vi "FRIC_navX_Internal_I2C_ProcessingLoop.vi"(7 "Device Number":T2, 10 "I2C Bus":T1=enum."I2C MXP", 11 "Rate (4Hz-200Hz)":u8=50 min=4 max=200) -> ()   [LabVIEW 2016]
doc: "This navX VI handles the reading/writing for the navX. All of the good stuff is in here.\nTHIS VI SHOULD NOT BE CALLED BY THE USER!"
uses:
  <vilib>/Rock Robotics/SystemInterfaces/i2clib/i2c_bus.ctl
  TypeDefs/Z900_navX_ProtocolTypeDef.ctl
  navX Library v2.lvlib
  TypeDefs/FRIC_navX_ProcessingLoopStatesTypeDef_I2C.ctl
  TypeDefs/Z900_navX_IntegrationControlRegisters.ctl
  TypeDefs/Z900_navX_ActionTypeDef.ctl
  TypeDefs/Z900_navX_NotifyPacketTypeDef.ctl
  TypeDefs/FRIC_navX_I2C Process Loop TypeDef.ctl
  TypeDefs/Flags/Z900_navX_Flags_CapabilityTypeDef.ctl
  TypeDefs/Z900_navX_DeviceRegisters.ctl
  <vilib>/Rock Robotics/SystemInterfaces/spilib/spi_bus.ctl
  <vilib>/Rock Robotics/WPI/SPI/WPI_SPIDevRef.ctl
  <vilib>/Rock Robotics/WPI/SerialPort/WPI_SerialPortRef.ctl
  TypeDefs/Z900_navX_SerialStreamTypeDef.ctl
  TypeDefs/FRIC_navX_DeviceNumbersTypeDef.ctl
  <vilib>/Rock Robotics/WPI/SerialPort/WPI_SerialPort.ctl
  <vilib>/Platform/TimedLoop/XDataNode/wakeup.ctl
  <vilib>/Platform/TimedLoop/XDataNode/XDNodeRunTimeDep.lvlib
  <vilib>/Platform/TimedLoop/XDataNode/nitl_modes.ctl
  <vilib>/Platform/TimedLoop/XDataNode/timing_clust.ctl
  <vilib>/Platform/TimedLoop/XDataNode/XDataNode.xnode
  <vilib>/ptbypt/NI_PtbyPt.lvlib
  TypeDefs/Z900_navX_DeviceTypeDef.ctl
panel:
  in  "Tab Control":enum32{"Page 1", "Page 2"}(tab)
  in  "Halt":bool
  out "Connected":bool
  out "error":errorcluster
  out "Loop Time":dbl
  out "Loop dt":i64
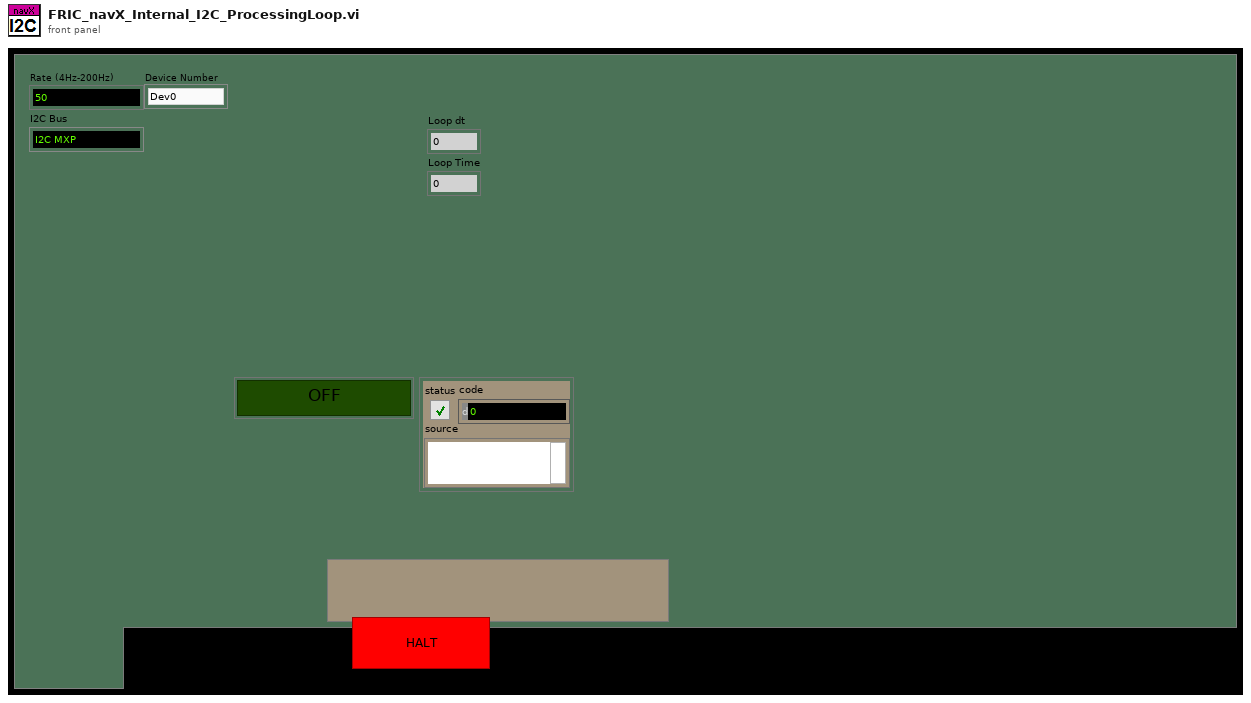
[diagram p1: front panel]
types:
  T1 = typedef "i2c_bus.ctl" = enum16{"I2C On-Board", "I2C MXP", "Invalid"}
  T2 = typedef "FRIC_navX_DeviceNumbersTypeDef.ctl" = enum16{"Dev0", "Dev1", "Dev2", "Dev3"}
  T3 = typedef "FRIC_navX_I2C Process Loop TypeDef.ctl" = cluster{"State Array":T4[], "error":errorcluster, "FPGA Cluster":cluster{"Last Valid FPGA Time":dbl, "Error Count":i32, "Initialized":bool}, "Device Info":T5, "I2CDevRef":cluster{"DevStatus":errorcluster, "Device Address":u8, "Handle":i32, "I2C Bus":T1}, "Registry":u8[], "Command Array":T7[], "Connected?":bool, "navX Device Memory Size":i32, "notification":T8, "Memory Size Set":bool, "SPIDevRef":T10, "navX Serial Open":cluster{"Stream Type":T12, "Serial Port":T13}, "SerialPortRef":T14, "Serial Read Buffer":string, "Serial Write Buffer":string[], "Device Number":T2, "navX SPI Open":cluster{"SPI Bus":T11, "Clock Rate (Hz)":dbl}, "Loop dt":i64, "current time":timestamp, "Loop Time":i64}
  T4 = typedef "FRIC_navX_ProcessingLoopStatesTypeDef_I2C.ctl" = enum16{"Process", "INI", "Check Packets Valid", "Close", "Flush Serial", "Generate Command", "Last Packet Valid", "Open", "Read", "Reset Serial", "Set Termination Char", "Update AE", "Wait", "Write", "Exit"}
  T5 = typedef "navX Library v2.lvlib/Z900_navX_DeviceTypeDef.ctl" = cluster{"Interface":cluster{"Protocol":T6, "Update Rate (4Hz-100Hz)":u8, "navX Open TypeDef":variant}, "Notify Packet":refnum<notifier>, "Loop VI Refnum":refnum<vi>, "Ready to Close Occurrence Refnum":refnum<k4>}
  T6 = typedef "navX Library v2.lvlib/Z900_navX_ProtocolTypeDef.ctl" = enum16{"SERIAL", "I2C", "SPI"}
  T7 = typedef "navX Library v2.lvlib/Z900_navX_IntegrationControlRegisters.ctl" = u8
  T8 = typedef "navX Library v2.lvlib/Z900_navX_NotifyPacketTypeDef.ctl" = cluster{"navX Action":T9, "Data":variant}
  T9 = typedef "navX Library v2.lvlib/Z900_navX_ActionTypeDef.ctl" = enum16{"None", "Halt", "Update Serial Protocol", "Zero-Yaw", "Zero-Displacement", "Zero-Velocity"}
  T10 = typedef "WPI_SPIDevRef.ctl" = cluster{"DevStatus":errorcluster, "Handle":i32, "SPI Bus":T11}
  T11 = typedef "spi_bus.ctl" = enum16{"SPI On-Board, CS0", "SPI On-Board, CS1", "SPI On-Board, CS2", "SPI On-Board, CS3", "SPI MXP", "Invalid"}
  T12 = typedef "navX Library v2.lvlib/Z900_navX_SerialStreamTypeDef.ctl" = enum16{"YRPH", "Quaterinons", "Gyro/Raw", "AHRS", "AHRSAndPositioning"}
  T13 = typedef "WPI_SerialPort.ctl" = enum16{"Onboard RS-232", "MXP TTL", "USB 1", "USB 2"}
  T14 = typedef "WPI_SerialPortRef.ctl" = cluster{"DevStatus":errorcluster, "Serial Port Name":refnum<visa-resource-name>}
  T15 = typedef "XDNodeRunTimeDep.lvlib/timing_clust.ctl" = cluster{"Expected End [f-1]":u64, "Actual End [f-1]":u64, "Finished Late? [f-1]":bool, "Expected End [i-1]":u64, "Actual End [i-1]":u64, "Finished Late? [i-1]":bool, "Expected Start [i]":u64, "Actual Start [i]":u64, "Expected Start [f]":u64, "Actual Start [f]":u64, "Source Name":string, "Structure Name":string, "Period":i64, "Deadline":i64, "Offset":i64, "Start":i64, "Priority":i32, "Timeout":i32, "Mode":T16, "Wakeup Reason":T17, "Error":errorcluster, "Source Type":string, "Secondary Source Type":string, "Global End Time":u64, "Global Start Time":u64, "Frame Duration":u64, "Iteration Duration":u64, "Assigned CPU":i32, "I/O Scan Engine Mode":u32}
  T16 = typedef "XDNodeRunTimeDep.lvlib/nitl_modes.ctl" = enum32{"No Change", "Process missed periods, maintain original phase", "Discard missed periods, maintain original phase", "Process missed periods, ignore original phase", "Discard missed periods, ignore original phase"}
  T17 = typedef "XDNodeRunTimeDep.lvlib/wakeup.ctl" = enum32{"Normal", "Aborted", "Asynchronous wakeup", "Timing source error", "Timed loop error", "Timeout"}
  T18 = typedef "Z900_navX_ActionTypeDef.ctl" = enum16{"None", "Halt", "Normal Read", "Update Serial Protocol", "Update Rate Htz", "Zero-Yaw", "Zero-Displacement", "Zero-Velocity"}
  T19 = typedef "navX Library v2.lvlib/Z900_navX_DeviceRegisters.ctl" = u8
  T20 = typedef "navX Library v2.lvlib/Z900_navX_Flags_CapabilityTypeDef.ctl" = u16
  T21 = cluster{"DevStatus":errorcluster, "Device Address":u8, "Handle":i32, "I2C Bus":T1}
  T22 = cluster{"Last Valid FPGA Time":dbl, "Error Count":i32, "Initialized":bool}
  T23 = typedef "WPI_I2CDevRef.ctl" = cluster{"DevStatus":errorcluster, "Device Address":u8, "Handle":i32, "I2C Bus":T1}
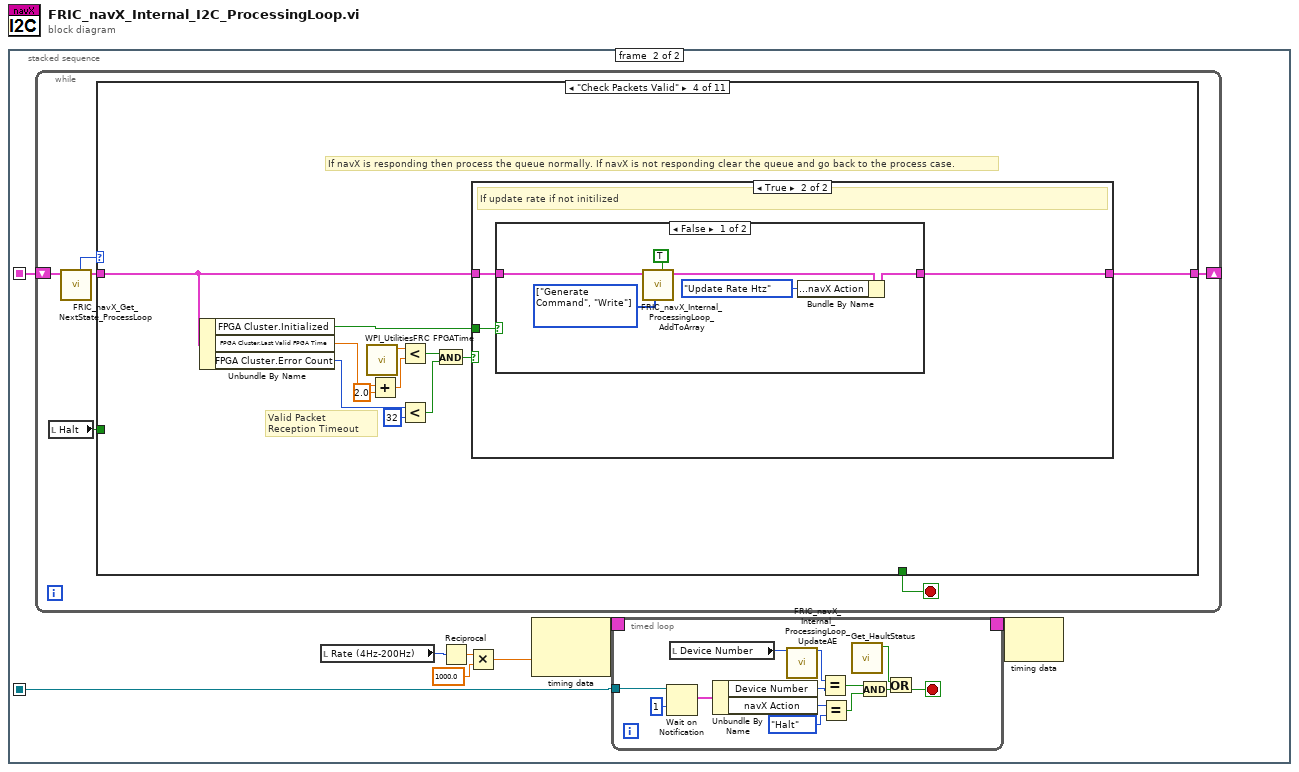
[diagram p0: block diagram]
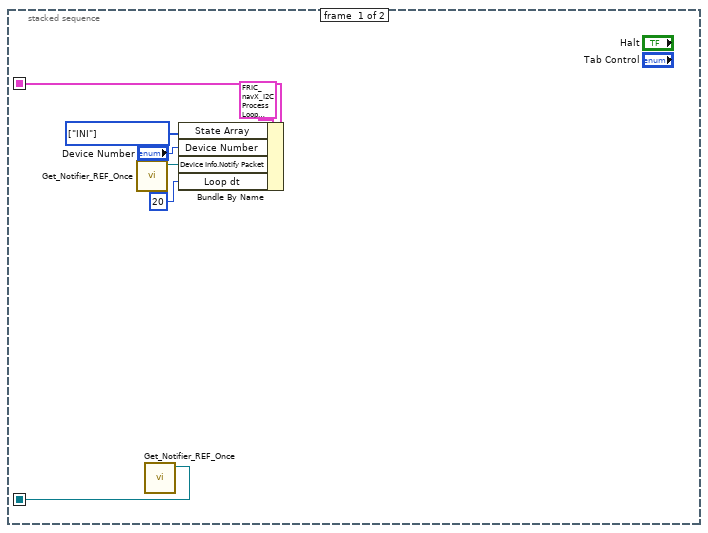
[diagram p2: hidden frame]
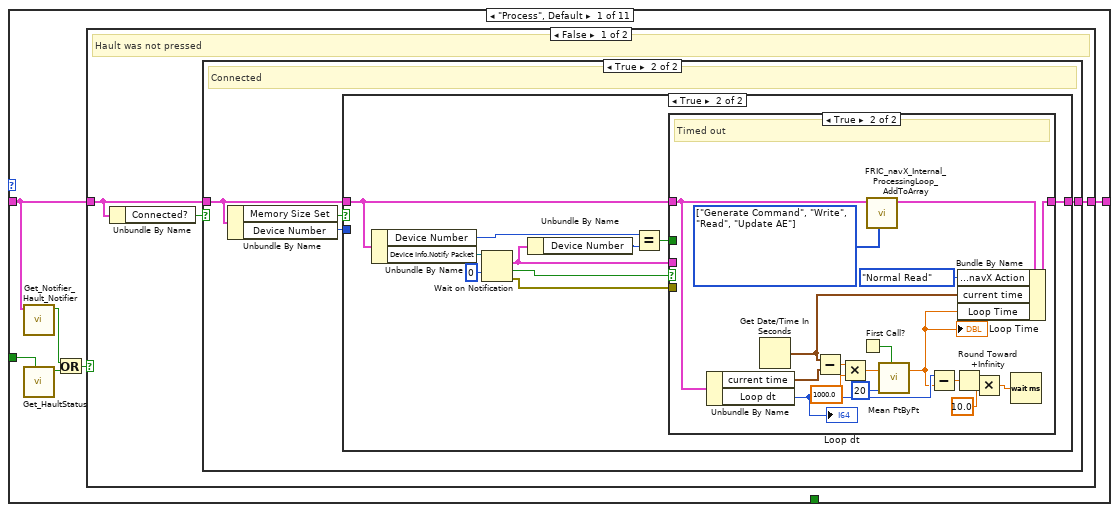
[diagram p3: hidden frame]
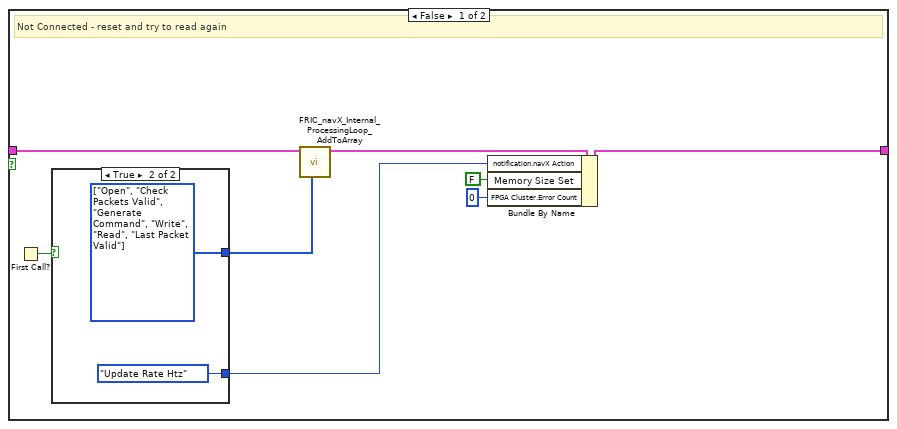
[diagram p4: hidden frame]
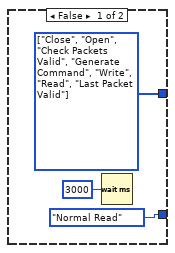
[diagram p5: hidden frame]
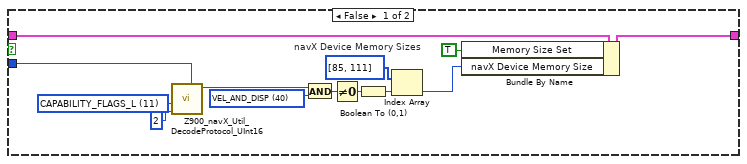
[diagram p6: hidden frame]
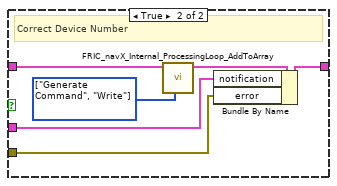
[diagram p8: hidden frame]
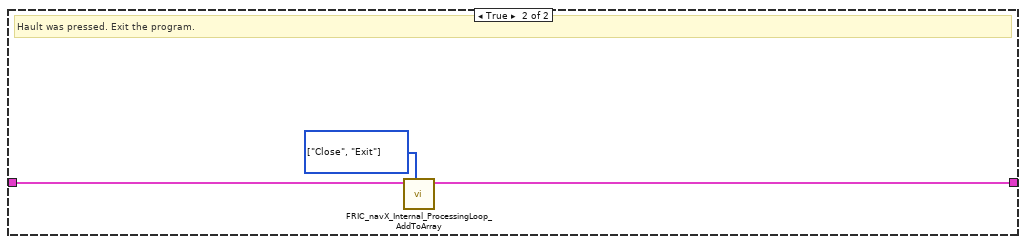
[diagram p9: hidden frame]
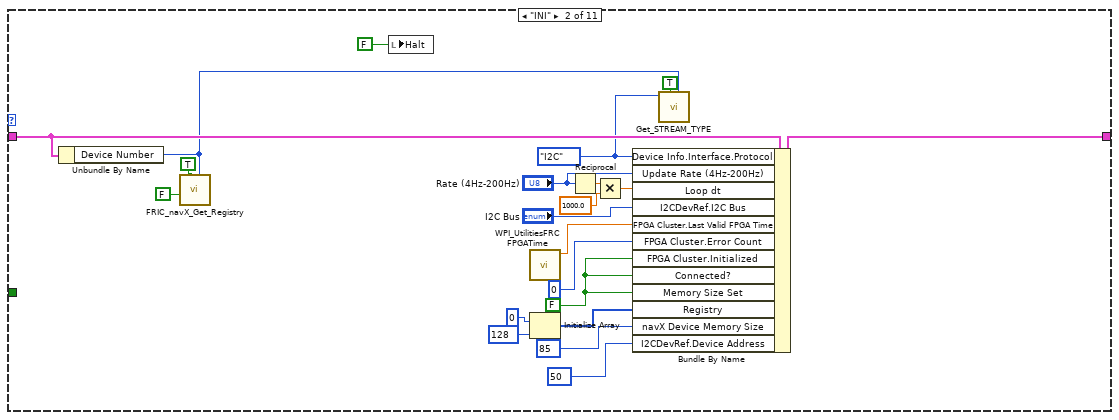
[diagram p10: hidden frame]
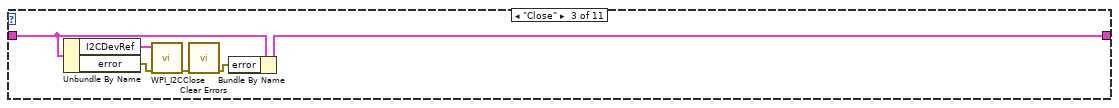
[diagram p11: hidden frame]
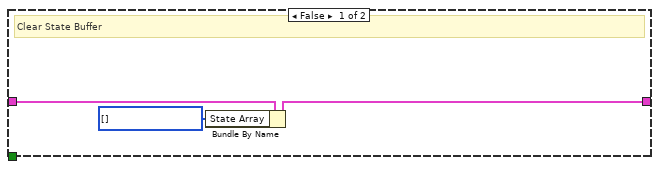
[diagram p12: hidden frame]
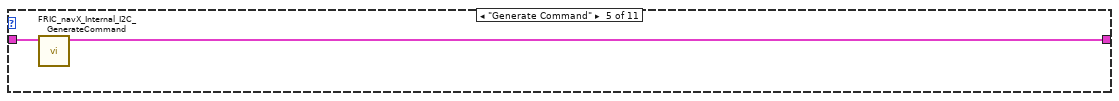
[diagram p14: hidden frame]
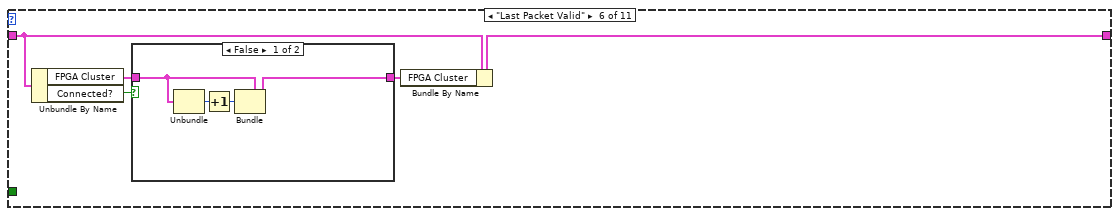
[diagram p15: hidden frame]
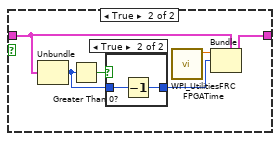
[diagram p16: hidden frame]
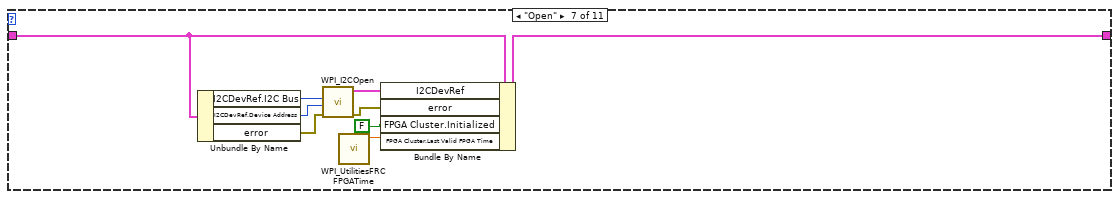
[diagram p18: hidden frame]
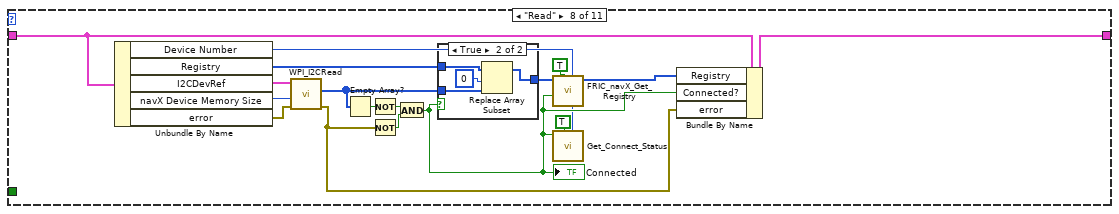
[diagram p19: hidden frame]
diagram:
  n1 = stacked-sequence {
    seq-local: [w7 _] -> [_ w15]
    seq-local: [w1 _] -> [_ w8]
    frame #0 {
      w5 = T4[] [enum."INI"] items=["Process", "INI", "Check Packets Valid", "Close", "Flush Serial", "Generate Command", "Last Packet Valid", "Open", "Read", "Reset Serial", "Set Termination Char", "Update AE", "Wait", "Write", "Exit"] ("State Array")
      n2 = call "Get_Notifier_REF_Once.vi"() -> ("notifier ref out"=w3:refnum<notifier>)  [unwired: 10 in, 1 out]
      n3 = call "Get_Notifier_REF_Once.vi"() -> ("notifier ref out"=w1:refnum<notifier>)  [unwired: 10 in, 1 out]
      n4 = Bundle By Name(cluster=T3 {"State Array"=[enum."INI", enum."Open"], "error"={"status"=FALSE, "code"=0, "source"=""}, "FPGA Cluster"={"Last Valid FPGA Time"=0.0, "Error Count"=0, "Initialized"=FALSE}, "Device Info"={"Interface"={"Protocol"=enum."SERIAL", "Update Rate (4Hz-100Hz)"=4, "navX Open TypeDef"=variant}, "Notify Packet"=refnum, "Loop VI Refnum"=refnum, "Ready to Close Occurrence Refnum"=refnum}, "I2CDevRef"={"DevStatus"={"status"=FALSE, "code"=0, "source"=""}, "Device Address"=0, "Handle"=0, "I2C Bus"=enum."Invalid"}, "Registry"=[], "Command Array"=[214, 32], "Connected?"=FALSE, "navX Device Memory Size"=85, "notification"={"navX Action"=enum."None", "Data"=variant}, "Memory Size Set"=FALSE, "SPIDevRef"={"DevStatus"={"status"=FALSE, "code"=0, "source"=""}, "Handle"=0, "SPI Bus"=enum."SPI On-Board, CS0"}, "navX Serial Open"={"Stream Type"=enum."YRPH", "Serial Port"=enum."Onboard RS-232"}, "SerialPortRef"={"DevStatus"={"status"=FALSE, "code"=0, "source"=""}, "Serial Port Name"=""}, "Serial Read Buffer"="", "Serial Write Buffer"=[], "Device Number"=enum."Dev0", "navX SPI Open"={"SPI Bus"=enum."SPI MXP", "Clock Rate (Hz)"=500000.0}, "Loop dt"=0, "current time"=timestamp(0 s since 1904-01-01), "Loop Time"=0} ("I2C Process Loop TypeDef"), "State Array"=w5, "Device Number"="Device Number", "Device Info.Notify Packet"=w3, "Loop dt"=i64 20) -> (w7:T3)
    }
    frame #1 {
      n5 = while {
        shift-right: [w35] -> _
        shift-left: w15 -> [w38]
        stop <- w39 stop-if-true
        n6 = local read "Halt"() -> (w34:bool)
        n7 = call "FRIC_navX_Get_NextState_ProcessLoop.vi"("I2C Process Loop TypeDef (in)"=w38) -> ("I2C Process Loop TypeDef (out)"=w37:T3, "Current State"=w36:T4)  [unwired: 9 in]
        n8 = case shown="\"Check Packets Valid\"" w36 {
          tunnel: [_ _ _ _ _ _ _ _ _ w233 _] -> w39
          tunnel: w37 -> [w44 w132 w146 w153 w175 w179 w201 w214 w231 w235 w243]
          tunnel: [w45 w138 w145 w154 w174 w178 w200 w213 w232 w235 w243] -> w35
          tunnel: w34 -> [w42 _ _ _ _ _ _ _ _ _ _]
          frame "Process", Default {
            n9 = call "Get_Notifier_Hault_Notifier.vi"("Process Loop TypeDef (in)"=w44) -> ("Hault Notifier"=w41:bool)  [unwired: 10 in]
            n10 = call "Get_HaultStatus.vi"("Update"=w42) -> ("Hault"=w40:bool)  [unwired: 10 in]
            n11 = Or(x=w41, y=w40) -> (x .or. y?=w43:bool)
            n12 = case shown="False" w43 {
              tunnel: [w48 w120] -> w45
              tunnel: w44 -> [w46 w121]
              frame False {
                # "Hault was not pressed"
                n13 = Unbundle By Name(w46) -> ("Connected?"=w47:bool)
                n14 = case shown="True" w47 {
                  tunnel: w46 -> [w56 w64]
                  tunnel: [w53 w65] -> w48
                  frame False {
                    # "Not Connected - reset and try to read again"
                    n15 = First Call?() -> (First Call?: T/F=w50:bool)
                    n16 = case shown="True" w50 {
                      tunnel: [w59 w61] -> w55
                      tunnel: [Z900_navX_ActionTypeDef."Normal Read" ("notification.navX Action") Z900_navX_ActionTypeDef."Update Rate Htz" ("notification.navX Action")] -> w49
                      frame False {
                        w59 = T4[] [enum."Close", enum."Open", enum."Check Packets Valid", enum."Generate Command", enum."Write", enum."Read", enum."Last Packet Valid"] items=["Process", "INI", "Check Packets Valid", "Close", "Flush Serial", "Generate Command", "Last Packet Valid", "Open", "Read", "Reset Serial", "Set Termination Char", "Update AE", "Wait", "Write", "Exit"]
                        n17 = Wait (ms)(milliseconds to wait=u32 3000) -> ()  [unwired: 1 out]
                      }
                      frame True {
                        w61 = T4[] [enum."Open", enum."Check Packets Valid", enum."Generate Command", enum."Write", enum."Read", enum."Last Packet Valid"] items=["Process", "INI", "Check Packets Valid", "Close", "Flush Serial", "Generate Command", "Last Packet Valid", "Open", "Read", "Reset Serial", "Set Termination Char", "Update AE", "Wait", "Write", "Exit"]
                      }
                    }
                    n18 = call "FRIC_navX_Internal_ProcessingLoop_AddToArray.vi"("States Array"=w55, "I2C Process Loop TypeDef (in)"=w56) -> ("I2C Process Loop TypeDef (out)"=w54:T3)  [unwired: 9 in]
                    n19 = Bundle By Name(cluster=w54, "notification.navX Action"=w49, "Memory Size Set"=FALSE, "FPGA Cluster.Error Count"=0) -> (w53:T3)
                  }
                  frame True {
                    # "Connected"
                    n20 = Unbundle By Name(w64) -> ("Memory Size Set"=w63:bool, "Device Number"=w62:T2)
                    n21 = case shown="True" w63 {
                      tunnel: [w77 w86] -> w65
                      tunnel: w64 -> [w78 w84]
                      tunnel: w62 -> [w66 _]
                      frame False {
                        w76 = T19 11 items=["WHOAMI"=0, "HW_REV"=1, "FW_VER_MAJOR"=2, "FW_VER_MINOR"=3, "UPDATE_RATE_HZ"=4, "ACCEL_FSR_G"=5, "GYRO_FSR_DPS"=6, "OP_STATUS"=8, "CAL_STATUS"=9, "SELFTEST_STATUS"=10, "CAPABILITY_FLAGS_L"=11, "CAPABILITY_FLAGS_H"=12, "SENSOR_STATUS"=16, "TIMESTAMP"=18, "YAW"=22, "ROLL"=24, "PITCH"=26, "HEADING"=28, "FUSED_HEADING"=30, "ALTITUDE_I"=32, "ALTITUDE_D"=34, "LINERA_ACC_X"=36, "LINERA_ACC_Y"=38, "LINERA_ACC_Z"=40, "QUAT_W"=42, "QUAT_X"=44, "QUAT_Y"=46, "QUAT_Z"=48, "MPU_TEMP_C"=50, "GYRO_X"=52, "GYRO_Y"=54, "GYRO_Z"=56, "ACC_X"=58, "ACC_Y"=60, "ACC_Z"=62, "MAG_X"=64, "MAG_Y"=66, "MAG_Z"=68, "PRESSURE_I"=70, "PRESSURE_D"=72, "PRESSURE_TEMP"=74, "YAW_OFFSET"=76, "QUAT_OFFSET_W"=78, "QUAT_OFFSET_X"=80, "QUAT_OFFSET_Y"=82, "QUAT_OFFSET_Z"=84, "INTEGRATION_CONTROL"=86, "VELOCITY_X"=88, "VELOCITY_Y"=92, "VELOCITY_Z"=96, "DISPLACMENT_X"=100, "DISPLACMENT_Y"=104, "DISPLACEMENT_Z"=108] ("Device Register")
                        w71 = T20 40 items=["OMNIMOUNT"=4, "OMNIMOUNT_CONFIG_MASK"=38, "VEL_AND_DISP"=40, "YAW_RESET"=80] ("Capability Flag")
                        w72 = i32[] [85, 111]  # navX Device Memory Sizes
                        n22 = call "Z900_navX_Util_DecodeProtocol_UInt16.vi"("Device Number"=w66, "length"=2, "Device Register"=w76) -> ("Value"=w69:u16)  [unwired: 8 in]
                        n23 = And(x=w69, y=w71) -> (x .and. y?=w70:T20)
                        n24 = Not Equal To 0?(x=w70) -> (x != 0?=w73:bool)
                        n25 = Boolean To (0,1)(Boolean=w73) -> (0, 1=w74:i16)
                        n26 = Index Array(array=w72, index=w74) -> (element=w68:i32)
                        n27 = Bundle By Name(cluster=w78, "Memory Size Set"=TRUE, "navX Device Memory Size"=w68) -> (w77:T3)
                      }
                      frame True {
                        n28 = Unbundle By Name(w84) -> ("Device Number"=w81:T2, "Device Info.Notify Packet"=w88:refnum<notifier>)
                        n29 = Wait on Notification(notifier=w88, timeout in ms (-1)=0) -> (notification=w82:T8, timed out?=w83:bool, error out=w85:errorcluster)  [unwired: 2 in, 1 out]
                        n30 = Unbundle By Name(w82) -> ("Device Number"=w80:T2)
                        n31 = Equal?(x=w81, y=w80) -> (x = y?=w79:bool)
                        n32 = case shown="True" w83 {
                          tunnel: w84 -> [w93 w114]
                          tunnel: [w92 w116] -> w86
                          tunnel: w82 -> [w91 _]
                          tunnel: w85 -> [w90 _]
                          tunnel: w79 -> [w89 _]
                          frame False {
                            # "Got a notifier"
                            n33 = case shown="False" w89 {
                              tunnel: w93 -> [w94 w100]
                              tunnel: [w94 w99] -> w92
                              tunnel: w91 -> [_ w98]
                              tunnel: w90 -> [_ w95]
                              frame False {
                              }
                              frame True {
                                w96 = T4[] [enum."Generate Command", enum."Write"] items=["Process", "INI", "Check Packets Valid", "Close", "Flush Serial", "Generate Command", "Last Packet Valid", "Open", "Read", "Reset Serial", "Set Termination Char", "Update AE", "Wait", "Write", "Exit"] ("States Array")
                                # "Correct Device Number"
                                n34 = call "FRIC_navX_Internal_ProcessingLoop_AddToArray.vi"("States Array"=w96, "I2C Process Loop TypeDef (in)"=w100) -> ("I2C Process Loop TypeDef (out)"=w97:T3)  [unwired: 9 in]
                                n35 = Bundle By Name(cluster=w97, "notification"=w98, "error"=w95) -> (w99:T3)
                              }
                            }
                          }
                          frame True {
                            w118 = T4[] [enum."Generate Command", enum."Write", enum."Read", enum."Update AE"] items=["Process", "INI", "Check Packets Valid", "Close", "Flush Serial", "Generate Command", "Last Packet Valid", "Open", "Read", "Reset Serial", "Set Termination Char", "Update AE", "Wait", "Write", "Exit"]
                            # "Timed out"
                            n36 = Unbundle By Name(w114) -> ("current time"=w112:timestamp, "Loop dt"=w109:i64)
                            "Loop dt" <- w109
                            n37 = Get Date/Time In Seconds() -> (seconds since 1Jan1904=w113:timestamp)
                            n38 = Subtract(x=w113, y=w112) -> (x-y=w111:dbl)
                            n39 = Multiply(x=w111, y=1000.0) -> (x*y=w108:dbl)
                            n40 = First Call?() -> (First Call?: T/F=w102:bool)
                            n41 = call "FRIC_navX_Internal_ProcessingLoop_AddToArray.vi"("States Array"=w118, "I2C Process Loop TypeDef (in)"=w114) -> ("I2C Process Loop TypeDef (out)"=w117:T3)  [unwired: 9 in]
                            n42 = call <vilib>:"Mean PtByPt.vi"("x"=w108, "sample length"=20, "initialize"=w102) -> ("mean"=w104:dbl)  [unwired: 1 in, 1 out]
                            "Loop Time" <- w104
                            n43 = Subtract(x=w109, y=w104) -> (x-y=w105:dbl)
                            n44 = Round Toward +Infinity(x=w105) -> (ceil(x): smallest int >= x=w107:dbl)
                            n45 = Bundle By Name(cluster=w117, "notification.navX Action"=Z900_navX_ActionTypeDef."Normal Read", "current time"=w113, "Loop Time"=w104) -> (w116:T3)
                            n46 = Multiply(x=w107, y=10.0) -> (x*y=w101:dbl)
                            n47 = Wait (ms)(milliseconds to wait=w101) -> ()  [unwired: 1 out]
                          }
                        }
                      }
                    }
                  }
                }
              }
              frame True {
                w119 = T4[] [enum."Close", enum."Exit"] items=["Process", "INI", "Check Packets Valid", "Close", "Flush Serial", "Generate Command", "Last Packet Valid", "Open", "Read", "Reset Serial", "Set Termination Char", "Update AE", "Wait", "Write", "Exit"] ("States Array")
                # "Hault was pressed. Exit the program."
                n48 = call "FRIC_navX_Internal_ProcessingLoop_AddToArray.vi"("States Array"=w119, "I2C Process Loop TypeDef (in)"=w121) -> ("I2C Process Loop TypeDef (out)"=w120:T3)  [unwired: 9 in]
              }
            }
          }
          frame "INI" {
            w122 = Z900_navX_ProtocolTypeDef."I2C" ("Protocol")
            w136 = FALSE ("Initialized")
            n49 = Unbundle By Name(w132) -> ("Device Number"=w123:T2)
            n50 = call "FRIC_navX_Get_Registry.vi"("Device Number"=w123, "Update"=TRUE, "Connected?"=FALSE) -> ()  [unwired: 7 in, 2 out]
            n51 = local write "Halt"(FALSE ("Halt")) -> ()
            n52 = call <vilib>:"WPI_UtilitiesFRC FPGATime.vi"() -> ("FPGA Time"=w140:dbl)  [unwired: 10 in, 1 out]
            n53 = Initialize Array(u8 0 ("Received Data"), 128 ("hex")) -> (w135:u8[])
            n54 = Reciprocal(x="Rate (4Hz-200Hz)") -> (1/x=w128:dbl)
            n55 = Multiply(x=w128, y=1000.0) -> (x*y=w127:dbl)
            n56 = Bundle By Name(cluster=w132, "Device Info.Interface.Protocol"=w122, "Update Rate (4Hz-200Hz)"="Rate (4Hz-200Hz)", "Loop dt"=w127, "I2CDevRef.I2C Bus"="I2C Bus", "FPGA Cluster.Last Valid FPGA Time"=w140, "FPGA Cluster.Error Count"=0 ("Error Count"), "FPGA Cluster.Initialized"=w136, "Connected?"=w136, "Memory Size Set"=w136, "Registry"=w135, "navX Device Memory Size"=85 ("hex"), "I2CDevRef.Device Address"=50 ("hex")) -> (w138:T3)
            n57 = call "Get_STREAM_TYPE.vi"("Device Number"=w123, "Update"=TRUE, "Protocol (in)"=w122) -> ()  [unwired: 8 in, 1 out]
          }
          frame "Close" {
            n58 = Unbundle By Name(w146) -> ("I2CDevRef"=w148:T21, "error"=w147:errorcluster)
            n59 = call <vilib>:"WPI_I2CClose.vi"("error in (no error)"=w147, "I2CDevRef"=w148) -> ("error out"=w144:errorcluster)  [unwired: 9 in]
            n60 = call <vilib>:"Clear Errors.vi"("error in (no error)"=w144) -> ("error out"=w143:errorcluster)  [unwired: 5 in, 1 out]
            n61 = Bundle By Name(cluster=w146, "error"=w143) -> (w145:T3)
          }
          frame "Check Packets Valid" {
            # "If navX is responding then process the queue normally. If navX is not responding clear the queue and go back to the process case."
            # "Valid Packet Reception Timeout"
            n62 = Unbundle By Name(w153) -> ("FPGA Cluster.Initialized"=w151:bool, "FPGA Cluster.Last Valid FPGA Time"=w152:dbl, "FPGA Cluster.Error Count"=w150:i32)
            n63 = call <vilib>:"WPI_UtilitiesFRC FPGATime.vi"() -> ("FPGA Time"=w158:dbl)  [unwired: 10 in, 1 out]
            n64 = Add(x=w152, y=2.0) -> (x+y=w159:dbl)
            n65 = Less?(x=w158, y=w159) -> (x < y?=w156:bool)
            n66 = Less?(x=w150, y=32) -> (x < y?=w155:bool)
            n67 = And(x=w156, y=w155) -> (x .and. y?=w149:bool)
            n68 = case shown="True" w149 {
              tunnel: w153 -> [w163 w166]
              tunnel: [w162 w165] -> w154
              tunnel: w151 -> [_ w164]
              frame False {
                w161 = T4[] [] items=["Process", "INI", "Check Packets Valid", "Close", "Flush Serial", "Generate Command", "Last Packet Valid", "Open", "Read", "Reset Serial", "Set Termination Char", "Update AE", "Wait", "Write", "Exit"] ("f")
                # "Clear State Buffer"
                n69 = Bundle By Name(cluster=w163, "State Array"=w161) -> (w162:T3)
              }
              frame True {
                # "If update rate if not initilized"
                n70 = case shown="False" w164 {
                  tunnel: w166 -> [w171 w173]
                  tunnel: [w169 w173] -> w165
                  frame False {
                    w167 = T4[] [enum."Generate Command", enum."Write"] items=["Process", "INI", "Check Packets Valid", "Close", "Flush Serial", "Generate Command", "Last Packet Valid", "Open", "Read", "Reset Serial", "Set Termination Char", "Update AE", "Wait", "Write", "Exit"] ("f")
                    n71 = call "FRIC_navX_Internal_ProcessingLoop_AddToArray.vi"("Add to beginning"=TRUE, "States Array"=w167, "I2C Process Loop TypeDef (in)"=w171) -> ("I2C Process Loop TypeDef (out)"=w170:T3)  [unwired: 8 in]
                    n72 = Bundle By Name(cluster=w170, "notification.navX Action"=Z900_navX_ActionTypeDef."Update Rate Htz") -> (w169:T3)
                  }
                  frame True {
                  }
                }
              }
            }
          }
          frame "Generate Command" {
            n73 = call "FRIC_navX_Internal_I2C_GenerateCommand.vi"("I2C Process Loop TypeDef (in)"=w175) -> ("I2C Process Loop TypeDef (out)"=w174:T3)  [unwired: 10 in]
          }
          frame "Last Packet Valid" {
            n74 = Unbundle By Name(w179) -> ("FPGA Cluster"=w180:T22, "Connected?"=w176:bool)
            n75 = case shown="False" w176 {
              tunnel: [w183 w190] -> w177
              tunnel: w180 -> [w182 w186]
              frame False {
                n76 = Unbundle(w182) -> ("Error Count"=w181:i32)  [unwired: 2 out]
                n77 = Increment(x=w181) -> (x+1=w184:i32)
                n78 = Bundle(cluster=w182, "Error Count"=w184) -> (w183:T22)  [unwired: 2 in]
              }
              frame True {
                n79 = Unbundle(w186) -> ("Error Count"=w185:i32)  [unwired: 2 out]
                n80 = Greater Than 0?(x=w185) -> (x > 0?=w188:bool)
                n81 = case shown="True" w188 {
                  tunnel: [w191 w193] -> w187
                  tunnel: w185 -> [w191 w192]
                  frame False {
                  }
                  frame True {
                    n82 = Decrement(x=w192) -> (x-1=w193:i32)
                  }
                }
                n83 = call <vilib>:"WPI_UtilitiesFRC FPGATime.vi"() -> ("FPGA Time"=w189:dbl)  [unwired: 10 in, 1 out]
                n84 = Bundle(cluster=w186, "Last Valid FPGA Time"=w189, "Error Count"=w187) -> (w190:T22)  [unwired: 1 in]
              }
            }
            n85 = Bundle By Name(cluster=w179, "FPGA Cluster"=w177) -> (w178:T3)
          }
          frame "Open" {
            n86 = Unbundle By Name(w201) -> ("I2CDevRef.I2C Bus"=w195:T1, "I2CDevRef.Device Address"=w194:u8, "error"=w196:errorcluster)
            n87 = call <vilib>:"WPI_I2COpen.vi"("error in"=w196, "Device Address"=w194, "I2C Bus"=w195) -> ("error out"=w199:errorcluster, "I2CDevRef"=w202:T23)  [unwired: 7 in]
            n88 = call <vilib>:"WPI_UtilitiesFRC FPGATime.vi"() -> ("FPGA Time"=w197:dbl)  [unwired: 10 in, 1 out]
            n89 = Bundle By Name(cluster=w201, "I2CDevRef"=w202, "error"=w199, "FPGA Cluster.Initialized"=FALSE ("Initialized"), "FPGA Cluster.Last Valid FPGA Time"=w197) -> (w200:T3)
          }
          frame "Read" {
            n90 = Unbundle By Name(w214) -> ("Device Number"=w206:T2, "Registry"=w203:u8[], "I2CDevRef"=w217:T21, "navX Device Memory Size"=w215:i32, "error"=w216:errorcluster)
            n91 = call <vilib>:"WPI_I2CRead.vi"("error in (no error)"=w216, "I2CBytesToRead"=w215, "I2CDevRef"=w217) -> ("error out"=w204:errorcluster, "Data Out"=w211:u8[])  [unwired: 6 in, 1 out]
            n92 = Empty Array?(array=w211) -> (empty?=w210:bool)
            n93 = Not(x=w210) -> (.not. x?=w209:bool)
            n94 = Not(x=w204) -> (.not. x?=w205:bool)
            n95 = And(x=w209, y=w205) -> (x .and. y?=w207:bool)
            "Connected" <- w207
            n96 = case shown="True" w207 {
              tunnel: w203 -> [w220 w224]
              tunnel: [w220 w223] -> w219
              tunnel: w211 -> [_ w222]
              frame False {
              }
              frame True {
                n97 = Replace Array Subset(array=w224, new element=w222, index=u8 0 ("hex")) -> (w223:u8[])
              }
            }
            n98 = call "FRIC_navX_Get_Registry.vi"("Device Number"=w206, "Update"=TRUE, "Connected?"=w207, "Registry (in)"=w219) -> ("Registry (out)"=w212:u8[])  [unwired: 6 in, 1 out]
            n99 = call "Get_Connect_Status.vi"("Device Number"=w206, "Update"=TRUE, "Connected"=w207) -> ()  [unwired: 8 in, 1 out]
            n100 = Bundle By Name(cluster=w214, "Registry"=w212, "Connected?"=w207, "error"=w204) -> (w213:T3)
          }
          frame "Write" {
            n101 = Unbundle By Name(w231) -> ("I2CDevRef"=w230:T21, "Command Array"=w228:T7[], "I2CDevRef.DevStatus"=w225:errorcluster)  [unwired: 1 out]
            n102 = Unbundle By Name(w230) -> ("Handle"=w227:i32, "Device Address"=w229:u8)
            n103 = call <vilib>:"i2clib_write.vi"("error in (no error)"=w225, "send_data"=w228, "dev_addr"=w229, "I2C Reference"=w227) -> ("error out"=w226:errorcluster)  [unwired: 6 in, 1 out]
            n104 = Bundle By Name(cluster=w231, "error"=w226) -> (w232:T3)
          }
          frame "Exit" {
            n105 = Unbundle By Name(w235) -> ("Device Info"=w234:T5)
            n106 = in-place {
              in-place-border: w234 -> [w238]
              in-place-border: [TRUE] -> w233
              # "Set Occurence of Close"
              n107 = Unbundle By Name(w238) -> ("Ready to Close Occurrence Refnum"=w239:refnum<k4>)
              n108 = local write "Halt"(FALSE ("Halt")) -> ()
              n109 = Set Occurrence(w239) -> ()
            }
          }
          frame "Update AE" {
            n110 = Unbundle By Name(w243) -> ("Device Number"=w241:T2, "error"=w242:errorcluster)
            "error" <- w242
            n111 = call "Get_Error_Status.vi"("Device Number"=w241, "Update"=TRUE, "error in"=w242) -> ()  [unwired: 8 in, 1 out]
          }
        }
      }
      n112 = local read "Rate (4Hz-200Hz)"() -> (w13:u8)
      n113 = Reciprocal(x=w13) -> (1/x=w14:dbl)
      n114 = Multiply(x=w14, y=1000.0) -> (x*y=w9:dbl)
      n115 = node-c288(w9) -> (w11:T15)  [unwired: 1 in]
      n116 = timed-loop {
        timing: w11 -> [_]
        timing-out: [_] -> w10
        tunnel: w8 -> [w24]
        stop <- w17 stop-if-true
        n117 = Wait on Notification(notifier=w24, timeout in ms (-1)=1) -> (notification=w23:T8)  [unwired: 2 in, 3 out]
        n118 = local read "Device Number"() -> (w21:T2)
        n119 = Unbundle By Name(w23) -> ("Device Number"=w22:T2, "navX Action"=w26:T9)
        n120 = call "FRIC_navX_Internal_ProcessingLoop_UpdateAE.vi"("Device Number"=w21) -> ()  [unwired: 15 in]
        n121 = Equal?(x=w21, y=w22) -> (x = y?=w20:bool)
        n122 = Equal?(x=w26, y=Z900_navX_ActionTypeDef."Halt") -> (x = y?=w19:bool)
        n123 = call "Get_HaultStatus.vi"() -> ("Hault"=w16:bool)  [unwired: 11 in]
        n124 = And(x=w20, y=w19) -> (x .and. y?=w18:bool)
        n125 = Or(x=w16, y=w18) -> (x .or. y?=w17:bool)
      }
      n126 = node-c288(w10) -> ()  [unwired: 1 out]
    }
  }
